vi "Start Countdown.vi"(8 "error in (no error)":errorcluster, 11 "Task Viewer in":refnum<class "Task Viewer.lvclass">) -> (0 "error out":errorcluster, 3 "Task Viewer out":refnum<class "Task Viewer.lvclass">)   [LabVIEW 2020, in "Task Viewer.lvlib" / "Task Viewer.lvclass"]
uses:
  Task Viewer.lvclass
  Task Viewer enum df.ctl
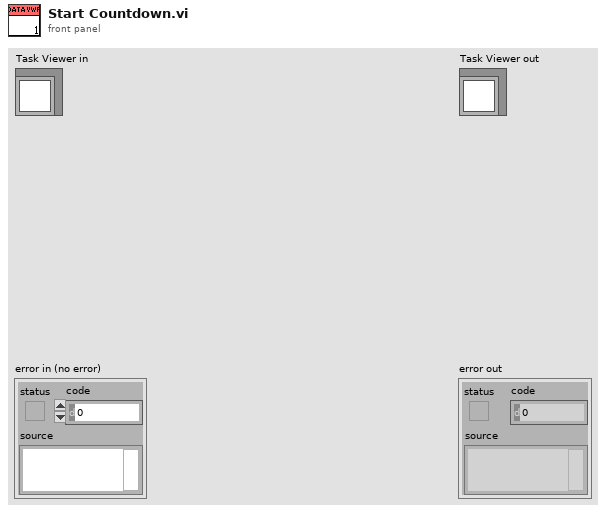
[diagram p1: front panel]
types:
  T1 = typedef "Task Viewer enum df.ctl" = enum16{"Idle", "Countdown", "Close Helper"}
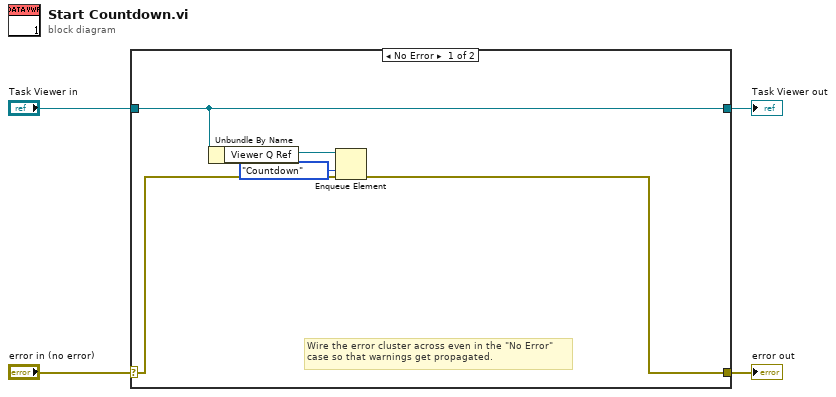
[diagram p0: block diagram]
diagram:
  n1 = case shown="No Error" "error in (no error)" {
    selector: "error in (no error)" -> [w7 w11]
    tunnel: [w6 w11] -> w3
    tunnel: [w9 w10] -> w1
    tunnel: "Task Viewer in" -> [w9 w10]
    frame No Error {
      # "Wire the error cluster across even in the \"No Error\"\ncase so that warnings get propagated."
      n2 = Unbundle By Name(w9) -> ("Viewer Q Ref"=w8:refnum<queue>)
      n3 = Enqueue Element(queue=w8, element=Task_Viewer_enum_df."Countdown", error in (no error)=w7) -> (error out=w6:errorcluster)  [unwired: 1 in, 2 out]
    }
    frame Error {
    }
  }
  "error out" <- w3
  "Task Viewer out" <- w1
